vi "To XML (Core).vi"(8 "error in (no error)":errorcluster, 10 "Parent":refnum<k20>, 11 "Test Suites in":refnum<class "Test Suites.lvclass">) -> (0 "error out":errorcluster)   [LabVIEW 2013, in "JUnit XML.lvlib" / "Test Suites.lvclass"]
doc: "Serializes Test Suites using NI XML Parser."
uses:
  Test Suites.lvclass
  JUnit XML.lvlib
  <vilib>/xml/NI_XML.lvlib
  <vilib>/xml/Close Reference(Node).vi
  Test Suite/Test Suite.lvclass
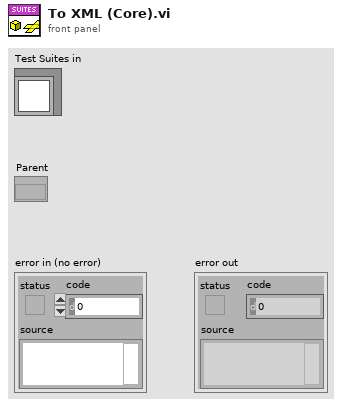
[diagram p1: front panel]
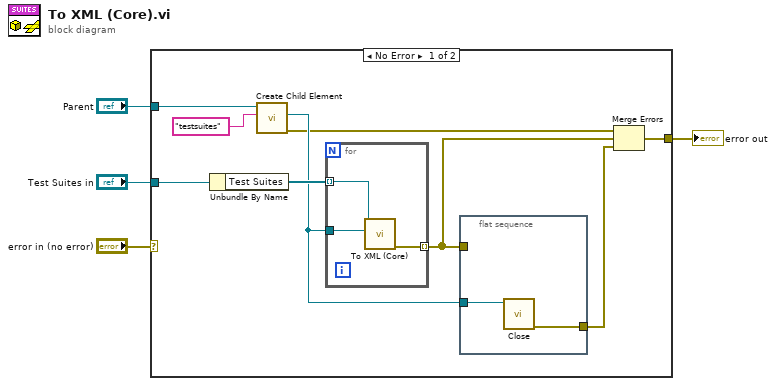
[diagram p0: block diagram]
diagram:
  n1 = case shown="No Error" "error in (no error)" {
    selector: "error in (no error)" -> [_ w19]
    tunnel: "Parent" -> [w13 _]
    tunnel: [w6 w19] -> w2
    tunnel: "Test Suites in" -> [w11 _]
    frame No Error {
      n2 = Unbundle By Name(w11) -> ("Test Suites"=w10:refnum<class "Test Suite.lvclass">[])
      n3 = call "Create Child Element.vi"("Name"="testsuites", "Node in"=w13) -> ("error out"=w8:errorcluster, "Child Element"=w9:refnum<k20>)  [unwired: 7 in, 1 out]
      n4 = for {
        tunnel: [w18] -> w5 mode=indexing
        tunnel: w10 -> [w17] mode=indexing
        tunnel: w9 -> [w16]
        n5 = call-dynamic "To XML (Core).vi"("Parent"=w16, "Test Suite in"=w17) -> ("error out"=w18:errorcluster)  [unwired: 9 in]
      }
      n6 = flat-sequence {
        tunnel: w9 -> [w15]
        tunnel: [w14] -> w7
        tunnel: w5 -> [_]
        frame #0 {
          n7 = call-poly <vilib>:"Close.vi"("node"=w15) -> ("error out"=w14:errorcluster)  [unwired: 8 in]
        }
      }
      n8 = Merge Errors(w8, w5, w7) -> (w6:errorcluster)
    }
    frame Error {
    }
  }
  "error out" <- w2
